vi "GetResponse.vi"(0 "Name":string, 1 "vi reference in":refnum<vi>) -> (2 "error out":errorcluster, 3 "value":string, 4 "All":cluster{"Name":string, "Variant Data":variant}[](array[cluster]), 5 "vi reference out":refnum<vi>)   [LabVIEW 2012]
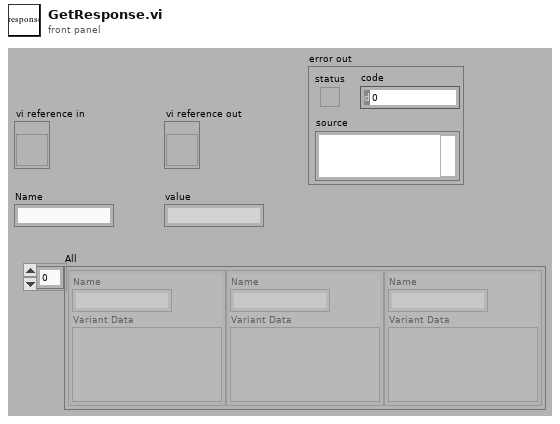
[diagram p1: front panel]
types:
  T1 = enum32{"Bad", "Idle", "Run top level", "Running"}
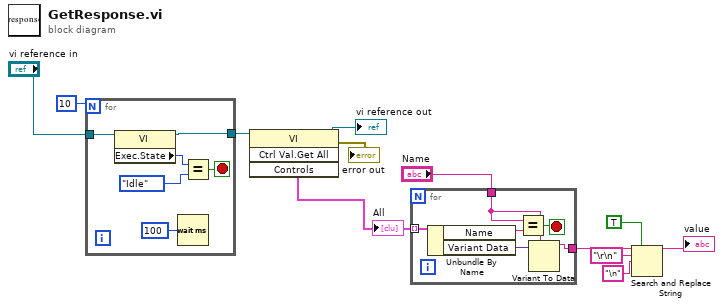
[diagram p0: block diagram]
diagram:
  n1 = for {
    N: 10 -> [_]
    tunnel: "vi reference in" -> [w18]
    tunnel: [w17] -> w7
    stop <- w14 stop-if-true
    n2 = property class="VI"(reference=w18) -> (reference out=w17:refnum<vi>, "Exec.State"=w16:T1)  [unwired: 1 in, 1 out]
    n3 = Wait (ms)(milliseconds to wait=u32 100) -> ()  [unwired: 1 out]
    n4 = Equal?(x=w16, y=T1."Idle" ("Execution:State")) -> (x = y?=w14:bool)
  }
  n5 = invoke class="VI" method="Ctrl Val.Get All"(reference=w7) -> (reference out=→"vi reference out":refnum<vi>, error out=→"error out":errorcluster, "Get All Control Values Variant"=w11:cluster{"Name":string, "Variant Data":variant}[])  [unwired: 3 in, 1 out]
  "All" <- w11
  n6 = for {
    tunnel: w11 -> [w24] mode=indexing
    tunnel: [w20] -> w4
    tunnel: "Name" -> [w19]
    stop <- w23 stop-if-true
    n7 = Unbundle By Name(w24) -> ("Name"=w22:string, "Variant Data"=w21:variant)
    n8 = Equal?(x=w19, y=w22) -> (x = y?=w23:bool)
    n9 = Variant To Data(type=w19, Variant=w21) -> (data=w20:string)  [unwired: 1 in, 1 out]
  }
  n10 = Search and Replace String(replace all?=TRUE ("replace all? (F)"), input string=w4, search string="\r\n", replace string="\n" ("search string")) -> (result string=→"value":string)  [unwired: 4 in, 3 out]
